vi "Set Vision Servo.vi"(8 "error in":errorcluster, 10 "Custom":i32, 11 "Setting":enum16{"Custom", "Boiler", "Gear"}(ring)=enum."Gear") -> (0 "error out":errorcluster)   [LabVIEW 2016, in "Vision Drive.lvlib"]
uses:
  Vision Drive.lvlib
  Constants/Private/Private Global.vi
  Constants/Constants.lvlib
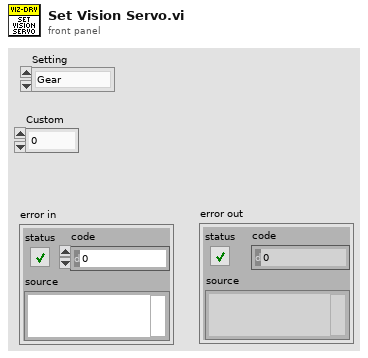
[diagram p1: front panel]
types:
  T1 = typedef "Constants.lvlib/Constants.ctl" = cluster{"Port Layout":cluster{"RightMotorInverted":bool, "LeftMotorInverted":bool, "Left Motors":T2, "Right Motors":T2, "Auton List":string[], "XBOX Port":T3, "Encoder L A":T4, "Encoder L B":T4, "Encoder R A":T4, "Encoder R B":T4, "L Encoder Inverse":bool, "R Encoder Inverse":bool, "Drive Distance per Count":dbl, "Gyro Bus":T5, "Fuel Roller 1":T2, "Front Roller":T2, "Gear Flipper":T2, "Climber 1":T2, "Fuel Roller Invert":bool, "Front Roller Invert":bool, "Gear Flipper Invert":bool, "Climber Invert":bool, "PCM":u8, "Fuel Roller 2":T2, "Gear Sensor":T6, "Gear Release Fwd":T7, "Gear Release Rvrs":T7, "Fuel Arm Fwd":T7, "Fuel Arm Rvrs":T7, "Shifter Fwrd":T7, "Shifter Rvrs":T7, "Climber 2":T2, "PDP":u8, "Shooter Front Channel":u8, "Shooter Rear Channel":u8, "Shooter Feed Channel":u8, "Camera Servo":T2, "Gear Servo":T2, "Gear Puncher Fwrd":T7, "Gear Puncher Rvrs":T7, "Shooter Inverse":bool, "Ring Light Switch":T4}, "Drive Constants":cluster{"Wheelbase In.":dbl, "Max Velocity (In/sec)":dbl, "Max Accel (In/sec^2)":dbl, "Max Jerk (In/sec^3)":dbl, "Path dt":dbl, "Path Sample Count":i32, "Deadband":dbl}, "Arm System":cluster{"Front Roller Gear Speed":dbl, "Front Roller Fuel Speed":dbl, "Gear Flipper Speed":dbl, "Fuel Roller Speed":dbl, "Gear Release Wait (ms)":i32, "Gear Sensor Threshold":dbl, "Flappy Open Angle":i32, "Flappy Close Angle":i32, "Ramp Rate (EGU/min)":dbl}, "Shooter":cluster{"Shooter Wheels":cluster{"P":dbl, "I":dbl, "D":dbl, "F":dbl, "IZone":dbl}, "Feeder":cluster{"P":dbl, "I":dbl, "D":dbl, "F":dbl, "IZone":dbl}, "Front Shooter RPM":dbl, "Rear Shooter RPM":dbl, "Agitator Speed":dbl, "Feeder Speed":dbl, "Shooter CPR":u32, "Feeder CPR":u32}, "Vision":cluster{"High Goal Height (in.)":dbl, "Low Goal Height (in.)":dbl, "Camera Height High (in.)":dbl, "Camera Height Low (in.)":dbl, "Servo Pitch Gear (deg)":dbl, "Camera Yaw (deg)":dbl, "Servo Gear":i32, "Servo Boiler":i32, "Servo Pitch Boiler (deg)":dbl}}
  T2 = typedef "FPGA_DIOPWMChannel.ctl" = enum8{"PWM 0", "PWM 1", "PWM 2", "PWM 3", "PWM 4", "PWM 5", "PWM 6", "PWM 7", "PWM 8", "PWM 9", "PWM MXP 0", "PWM MXP 1", "PWM MXP 2", "PWM MXP 3", "PWM MXP 4", "PWM MXP 5", "PWM MXP 6", "PWM MXP 7", "PWM MXP 8", "PWM MXP 9", "Invalid"}
  T3 = typedef "WPI_JoystickDeviceEnum.ctl" = enum16{"USB 0", "USB 1", "USB 2", "USB 3", "USB 4", "USB 5"}
  T4 = typedef "FPGA_DIOChannel.ctl" = enum8{"DIO 0", "DIO 1", "DIO 2", "DIO 3", "DIO 4", "DIO 5", "DIO 6", "DIO 7", "DIO 8", "DIO 9", "DIO MXP 0", "DIO MXP 1", "DIO MXP 2", "DIO MXP 3", "DIO MXP 4", "DIO MXP 5", "DIO MXP 6", "DIO MXP 7", "DIO MXP 8", "DIO MXP 9", "DIO MXP 10", "DIO MXP 11", "DIO MXP 12", "DIO MXP 13", "DIO MXP 14", "DIO MXP 15", "SPI Port CS1", "SPI Port CS2", "SPI Port CS3", "SPI Port MISO", "SPI Port MOSI", "Invalid"}
  T5 = typedef "spi_bus.ctl" = enum16{"SPI On-Board, CS0", "SPI On-Board, CS1", "SPI On-Board, CS2", "SPI On-Board, CS3", "SPI MXP", "Invalid"}
  T6 = typedef "FPGA_AIChannel.ctl" = enum8{"AI 0", "AI 1", "AI 2", "AI 3", "AI MXP 0", "AI MXP 1", "AI MXP 2", "AI MXP 3", "Invalid"}
  T7 = typedef "WPI_SolenoidChannel.ctl" = enum8{"Solenoid 0", "Solenoid 1", "Solenoid 2", "Solenoid 3", "Solenoid 4", "Solenoid 5", "Solenoid 6", "Solenoid 7", "Invalid"}
  T8 = typedef "WPI_ServoDeviceRef.ctl" = cluster{"DeviceStatus":errorcluster, "PWM Channel":T2, "DeadBand":T9}
  T9 = typedef "WPI_PWMDeadband.ctl" = cluster{"Name":string, "maxPositivePwm":i32, "minPositivePwm":i32, "centerPwm":i32, "maxNegativePwm":i32, "minNegativePwm":i32, "angularRange":u16}
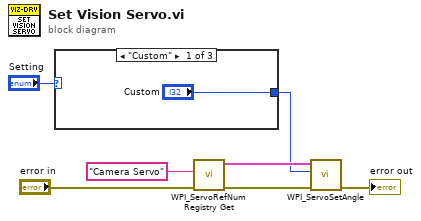
[diagram p0: block diagram]
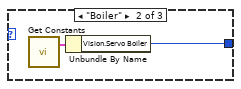
[diagram p2: hidden frame]
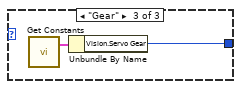
[diagram p3: hidden frame]
diagram:
  n1 = case shown="\"Custom\"" "Setting" {
    tunnel: ["Custom" w9 w11] -> w1
    frame "Custom" {
    }
    frame "Boiler" {
      n2 = call "Get Constants.vi"() -> ("Constants"=w10:T1)  [unwired: 3 in]
      n3 = Unbundle By Name(w10) -> ("Vision.Servo Boiler"=w9:i32)
    }
    frame "Gear" {
      n4 = call "Get Constants.vi"() -> ("Constants"=w12:T1)  [unwired: 3 in]
      n5 = Unbundle By Name(w12) -> ("Vision.Servo Gear"=w11:i32)
    }
  }
  n6 = call <vilib>:"WPI_ServoRefNum Registry Get.vi"("error in (no error)"="error in", "refnum name"="Camera Servo") -> ("error out"=w5:errorcluster, "ServoDeviceRef"=w6:T8)  [unwired: 8 in]
  n7 = call <vilib>:"WPI_ServoSetAngle.vi"("error in (no error)"=w5, "Angle"=w1, "ServoDeviceRef"=w6) -> ("error out"=→"error out":errorcluster)  [unwired: 7 in, 1 out]
